vi "Untitled 1.vi"() -> ()   [LabVIEW 2010]
panel:
  out "dataout":string
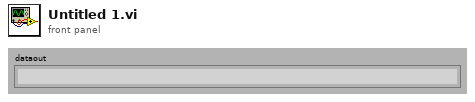
[diagram p1: front panel]
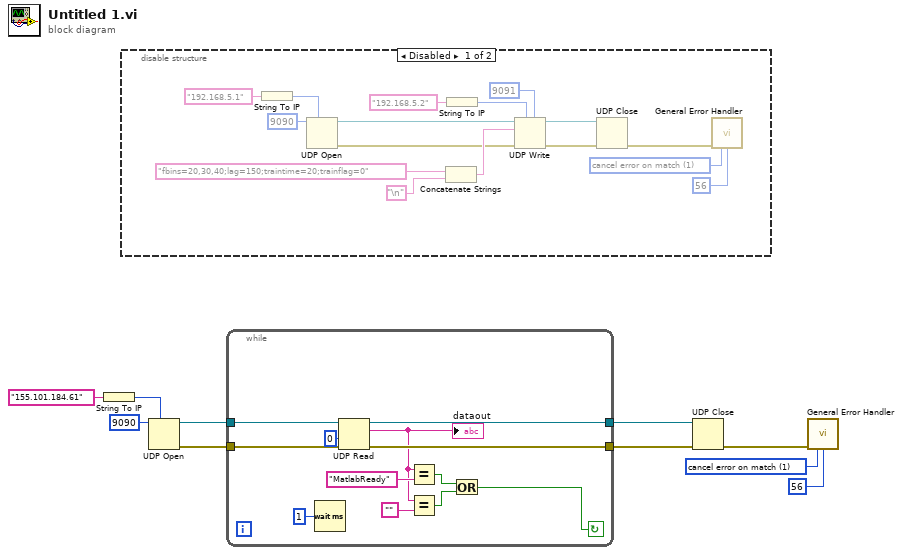
[diagram p0: block diagram]
diagram:
  w4 = 1 items=["no exception", "cancel error on match", "set error on match"] ("[exception action] (none:0)")
  n1 = String To IP(1:"155.101.184.61" ("name")) -> (0:w6:u32)
  n2 = disable-structure shown="Disabled" {
    frame Disabled {
      w15 = 1 items=["no exception", "cancel error on match", "set error on match"] ("[exception action] (none:0)")
      n3 = String To IP(1:"192.168.5.1" ("name")) -> (0:w21:u32)
      n4 = UDP Open(7:w21, 11:u16 9090 ("port")) -> (port=w20:refnum<k16>, 0:w12:errorcluster)  [unwired: 3 in, 1 out]
      n5 = Concatenate Strings("fbins=20,30,40;lag=150;traintime=20;trainflag=0" ("data in"), "\n") -> (w17:string)
      n6 = String To IP(1:"192.168.5.2" ("name")) -> (0:w25:u32)
      n7 = UDP Write(address=w25, port or service name=u16 9091 ("port"), connection ID=w20, data in=w17, 8:w12) -> (error out=w13:errorcluster, 3:w11:refnum<k16>)  [unwired: 1 in]
      n8 = UDP Close(connection ID=w11, 8:w13) -> (error out=w14:errorcluster)  [unwired: 1 out]
      n9 = call <vilib>:"General Error Handler.vi"("error in (no error)"=w14, "[exception action] (none:0)"=w15, "[exception code]"=56) -> ()  [unwired: 8 in, 5 out]
    }
    frame Enabled {
    }
  }
  n10 = UDP Open(7:w6, 11:u16 9090 ("port")) -> (port=w9:refnum<k16>, 0:w10:errorcluster)  [unwired: 3 in, 1 out]
  n11 = while {
    tunnel: w10 -> [w37]
    tunnel: w9 -> [w36]
    tunnel: [w35] -> w2
    tunnel: [w34] -> w1
    stop <- w28 continue-if-true
    n12 = Wait (ms)(milliseconds to wait=u32 1) -> ()  [unwired: 1 out]
    n13 = UDP Read(connection ID=w36, timeout ms (25000)=0, 8:w37) -> (data out=w31:string, error out=w34:errorcluster, 3:w35:refnum<k16>)  [unwired: 1 in, 2 out]
    "dataout" <- w31
    n14 = Equal?(x=w31, y="MatlabReady") -> (x = y?=w30:bool)
    n15 = Equal?(x=w31, y="") -> (x = y?=w29:bool)
    n16 = Or(x=w30, y=w29) -> (x .or. y?=w28:bool)
  }
  n17 = UDP Close(connection ID=w2, 8:w1) -> (error out=w3:errorcluster)  [unwired: 1 out]
  n18 = call <vilib>:"General Error Handler.vi"("error in (no error)"=w3, "[exception action] (none:0)"=w4, "[exception code]"=56) -> ()  [unwired: 8 in, 5 out]
